vi "Write Temp.vi"(7 "target":dbl caption="Target Temp") -> (1 "temp":dbl caption="Temperature", 2 "tempdiff>60":bool caption="Temp Diff > 60", 3 "targetOUT":dbl caption="Target Temp")   [LabVIEW 2009, in "Magnet.lvclass"]
uses:
  Magnet.lvclass
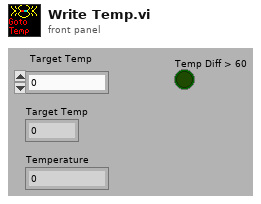
[diagram p1: front panel]
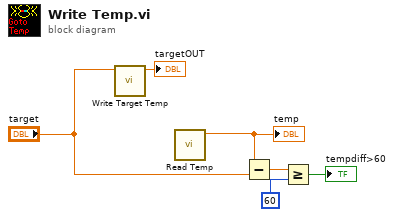
[diagram p0: block diagram]
diagram:
  n1 = call "Write Target Temp.vi"("target"="target") -> ("targetOUT"=→"targetOUT":dbl)  [unwired: 6 out]
  n2 = call "Read Temp.vi"() -> ("temp"=w2:dbl)  [unwired: 7 out]
  "temp" <- w2
  n3 = Subtract(x=w2, y="target") -> (x-y=w6:dbl)
  n4 = Greater Or Equal?(x=w6, y=60) -> (x >= y?=→"tempdiff>60":bool)
